vi "Lakeshore 336 Set Parameters GUI.vi"(10 "Lakeshore 336 Settings.Input Ch":T1[](array[typedef]), 11 "Lakeshore 336 Settings.Output Ch":T2[](array[typedef]) {"Heater Resistance (1:25 Ohms)" items=["25 Ohms"=1, "50 Ohms"=2]; "Max User Current (2.000)" format="%.3f"; "Heater Out Display (1:Current)" items=["Current"=1, "Power"=2]; "Max Current (0:User Specified)" items=["User Specified", "0.707 A", "1.0 A", "1.141 A", "2.0 A"]; "Mode (0:Off)" items=["Off", "Closed Loop PID", "Zone", "Open Loop"]; "Input (0:None)" items=["None", "A", "B", "C", "D"]}) -> (1 "Cancelled":bool, 2 "Lakeshore 336 Settings.Input Ch out":T1[](array[typedef]), 3 "Lakeshore 336 Settings.Output Ch":T2[](array[typedef]) {"Heater Resistance (1:25 Ohms)" items=["25 Ohms"=1, "50 Ohms"=2]; "Max User Current (2.000)" format="%.3f"; "Heater Out Display (1:Current)" items=["Current"=1, "Power"=2]; "Max Current (0:User Specified)" items=["User Specified", "0.707 A", "1.0 A", "1.141 A", "2.0 A"]; "Mode (0:Off)" items=["Off", "Closed Loop PID", "Zone", "Open Loop"]; "Input (0:None)" items=["None", "A", "B", "C", "D"]})   [LabVIEW 2022 SP3, in "Lakeshore 336.lvclass"]
uses:
  Lakeshore 336.lvclass
  Lakeshore 336 Channel Settings cluster.ctl
  Lakeshore 336 PID cluster.ctl
  Lakeshore 336 Input Ch config cluster.ctl
  Lakeshore 336.lvclass/Lakeshore 336.ctl
panel:
  in  "OK Button":bool
  in  "Cancel Button":bool
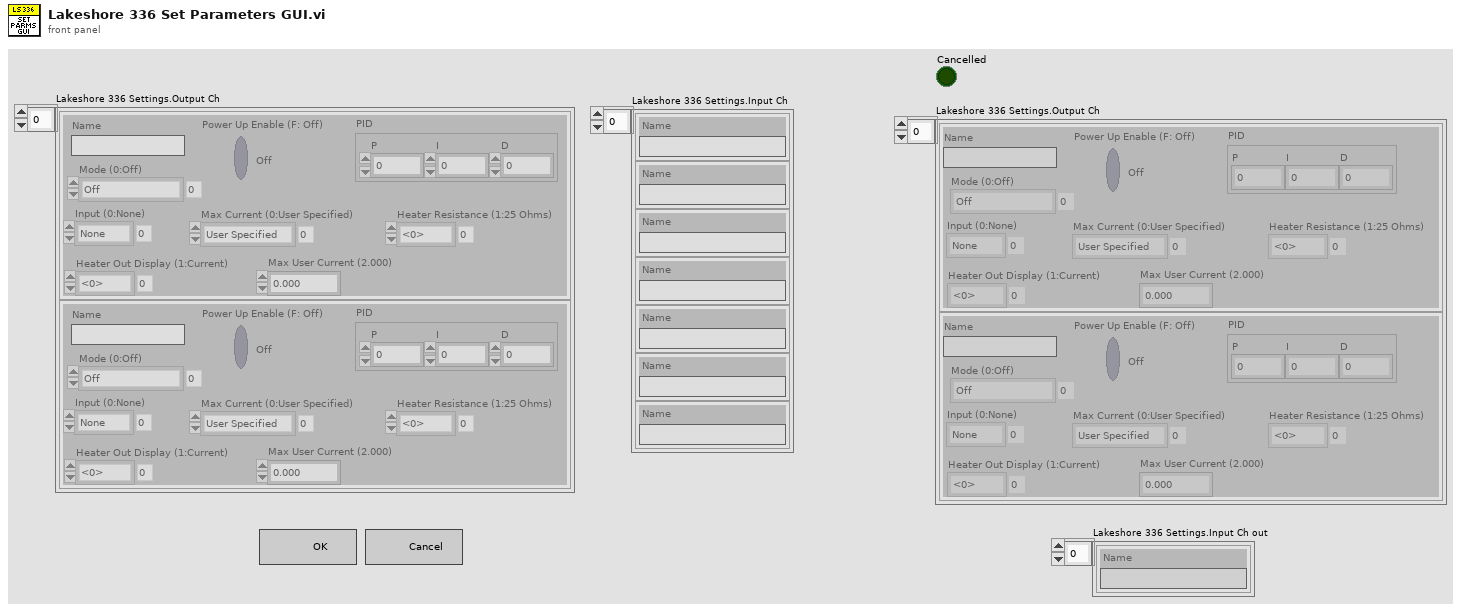
[diagram p1: front panel]
types:
  T1 = typedef "Lakeshore 336.lvclass/Lakeshore 336 Input Ch config cluster.ctl" = cluster{"Name":string}
  T2 = typedef "Lakeshore 336.lvclass/Lakeshore 336 Channel Settings cluster.ctl" = cluster{"Input (0:None)":u16, "Power Up Enable (F: Off)":bool, "Mode (0:Off)":u16, "Max Current (0:User Specified)":u16, "Heater Out Display (1:Current)":u16, "Max User Current (2.000)":dbl, "Heater Resistance (1:25 Ohms)":u16, "PID":T3, "Name":string}
  T3 = typedef "Lakeshore 336.lvclass/Lakeshore 336 PID cluster.ctl" = cluster{"P":dbl, "I":dbl, "D":dbl}
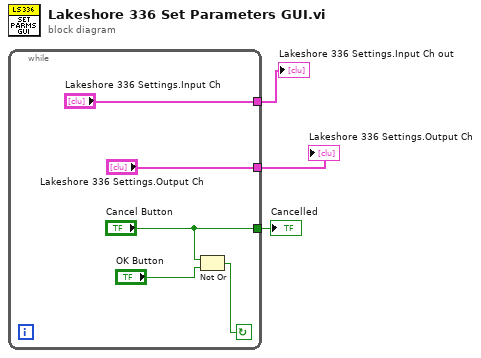
[diagram p0: block diagram]
diagram:
  n1 = while {
    tunnel: ["Lakeshore 336 Settings.Output Ch"] -> w1
    tunnel: ["Cancel Button"] -> w3
    tunnel: ["Lakeshore 336 Settings.Input Ch"] -> w2
    stop <- w6 continue-if-true
    n2 = Not Or(1:"OK Button", 2:"Cancel Button") -> (0:w6:bool)
  }
  "Lakeshore 336 Settings.Output Ch" <- w1
  "Cancelled" <- w3
  "Lakeshore 336 Settings.Input Ch out" <- w2
